vi "写入数值.vi"(8 "error in (no error)":errorcluster caption="错误输入（无错误）", 10 "数值":dbl, 11 "DATA输入":refnum<class "DATA.lvclass">) -> (0 "error out":errorcluster caption="错误输出", 3 "DATA输出":refnum<class "DATA.lvclass">)   [LabVIEW 2011, in "List.lvlib" / "DATA.lvclass"]
uses:
  DATA.lvclass
  DATA.lvclass/DATA.ctl
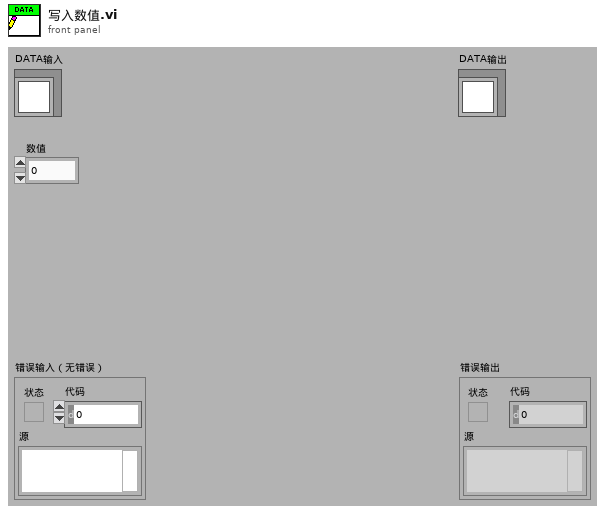
[diagram p1: front panel]
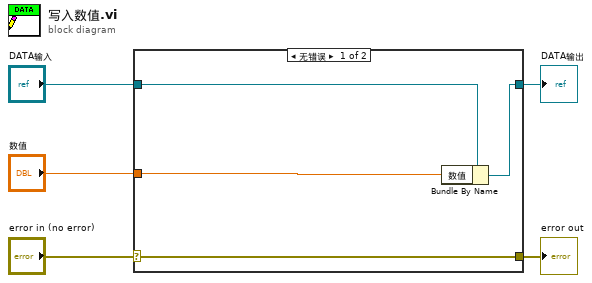
[diagram p0: block diagram]
diagram:
  n1 = case shown="无错误" "error in (no error)" {
    selector: "error in (no error)" -> [w9 w10]
    tunnel: [w9 w10] -> w4
    tunnel: [w7 w11] -> w2
    tunnel: "DATA输入" -> [w8 w11]
    tunnel: "数值" -> [w6 _]
    frame No Error {
      n2 = Bundle By Name(cluster=w8, "数值"=w6) -> (w7:refnum<class "DATA.lvclass">)
    }
    frame Error {
    }
  }
  "error out" <- w4
  "DATA输出" <- w2
